vi "BGImage.vi"(9 "index":i32, 10 "BG":T1, 11 "Image":T1) -> (3 "Refnum out":T1, 4 "time":u32)   [LabVIEW 2011, in "MagAnalysis_Online.lvclass"]
uses:
  MagAnalysis_Online.lvclass
  IMAQ Image.ctl
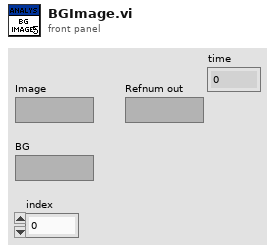
[diagram p1: front panel]
types:
  T1 = typedef "IMAQ Image.ctl" = refnum<image>
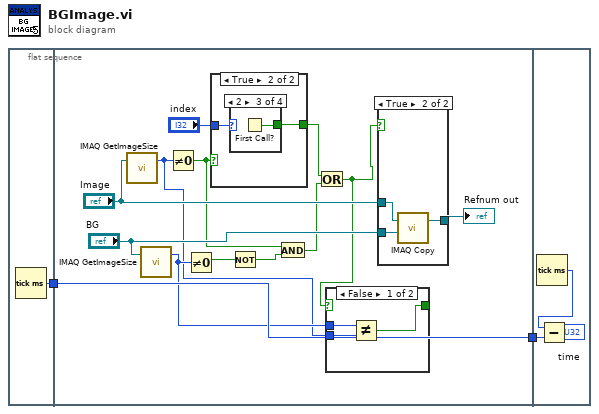
[diagram p0: block diagram]
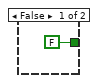
[diagram p3: hidden frame]
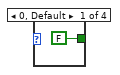
[diagram p4: hidden frame]
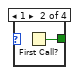
[diagram p5: hidden frame]
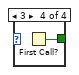
[diagram p6: hidden frame]
diagram:
  n1 = flat-sequence {
    tunnel: [w3] -> w2
    tunnel: w2 -> [w13]
    tunnel: [w13] -> w1
    tunnel: w1 -> [w33]
    frame #0 {
      n2 = Tick Count (ms)() -> (millisecond timer value=w3:u32)
    }
    frame #1 {
      n3 = call "IMAQ GetImageSize"("Image"="Image") -> ("Y Resolution"=w5:i32)  [unwired: 3 in, 2 out]
      n4 = call "IMAQ GetImageSize"("Image"="BG") -> ("Y Resolution"=w6:i32)  [unwired: 3 in, 2 out]
      n5 = Not Equal To 0?(x=w5) -> (x != 0?=w8:bool)
      n6 = Not Equal To 0?(x=w6) -> (x != 0?=w10:bool)
      n7 = case shown="True" w8 {
        tunnel: [FALSE ("First Call?: T/F") w23] -> w12
        tunnel: "index" -> [_ w22]
        frame False {
        }
        frame True {
          n8 = case shown="2" w22 {
            tunnel: [FALSE ("First Call?: T/F") w25 w26 w27] -> w23
            frame 0, Default {
            }
            frame 1 {
              n9 = First Call?() -> (First Call?: T/F=w25:bool)
            }
            frame 2 {
              n10 = First Call?() -> (First Call?: T/F=w26:bool)
            }
            frame 3 {
              n11 = First Call?() -> (First Call?: T/F=w27:bool)
            }
          }
        }
      }
      n12 = Not(x=w10) -> (.not. x?=w9:bool)
      n13 = And(x=w8, y=w9) -> (x .and. y?=w7:bool)
      n14 = Or(x=w12, y=w7) -> (x .or. y?=w4:bool)
      n15 = case shown="False" w4 {
        selector: w4 -> [_ w20]
        tunnel: w6 -> [w19 _]
        tunnel: w5 -> [w18 _]
        tunnel: [w17 w20] -> _
        frame False {
          n16 = Not Equal?(x=w19, y=w18) -> (x != y?=w17:bool)
        }
        frame True {
        }
      }
      n17 = case shown="True" w4 {
        tunnel: [w28 w29] -> w15
        tunnel: "BG" -> [w28 w31]
        tunnel: "Image" -> [_ w30]
        frame False {
        }
        frame True {
          n18 = call "IMAQ Copy"("Image Dst"=w31, "Image Src"=w30) -> ("Image Dst Out"=w29:T1)  [unwired: 4 in, 1 out]
        }
      }
      "Refnum out" <- w15
    }
    frame #2 {
      n19 = Tick Count (ms)() -> (millisecond timer value=w34:u32)
      n20 = Subtract(x=w34, y=w33) -> (x-y=→"time":u32)
    }
  }
